vi "Global_ACT_Data Out.vi"() -> ()   [LabVIEW 2020, in "SwerveDrive_ACT_ts.lvlib"]
uses:
  SwerveDrive_ACT_ts.lvlib
panel:
  in  "ACT_SwerveDrive_Speeds":dbl[](array[numeric])
  in  "ACT_Template_CycleTime(S)":dbl
  in  "ACT_SwerveDrive_Directions":dbl[](array[numeric])
  # "The Names of the Data items in the Global Variable MUST describe who the Single Writer is\nFor Actuator Globals the the naming convention is\n   \nACT_Lib Name_Data Name\n\nExamples:\nACT_Drive_X axis\nACT_Hopper_AgitatorSpeed"
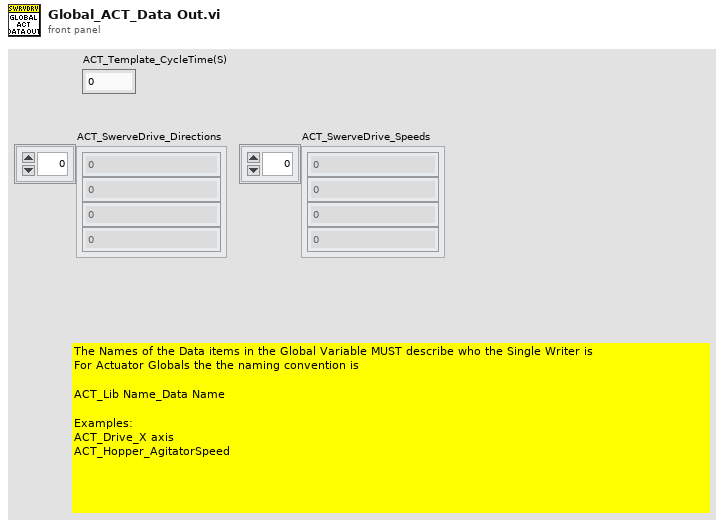
[diagram p1: front panel]
diagram:
